vi "vision board process.vi"(11 "Array in":string[][](array[string])) -> (3 "Array out":string[][](array[string]))   [LabVIEW 2019]
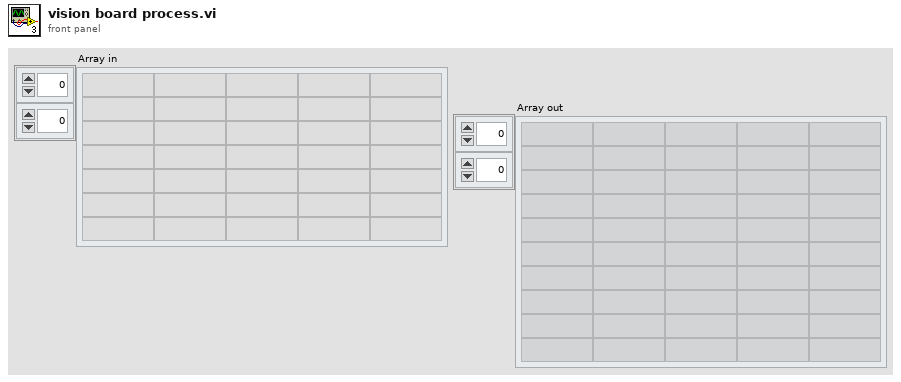
[diagram p1: front panel]
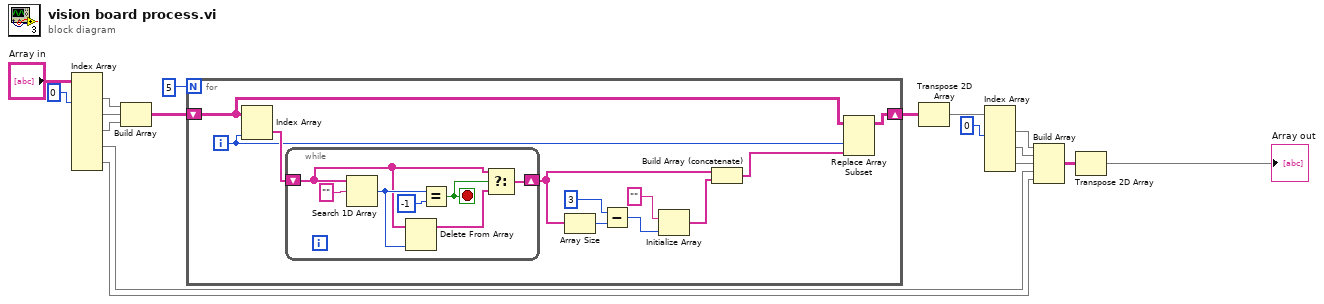
[diagram p0: block diagram]
diagram:
  n1 = Index Array(array="Array in", index (col) #1=0 ("disabled index (col)")) -> (element #1=w1:string[], element #2=w3:string[], element #3=w2:string[], element #4=w13:string[], element #5=w12:string[])  [unwired: 9 in]
  n2 = Build Array(w1, w3, w2) -> (w6:string[][])
  n3 = for {
    N: 5 -> [_]
    shift-right: [w28] -> w11
    shift-left: w6 -> [w26]
    i -> [w25]
    n4 = Index Array(array=w26, index (col)=w25) -> (element=w27:string[])  [unwired: 1 in]
    n5 = while {
      shift-right: [w29] -> w19
      shift-left: w27 -> [w30]
      stop <- w31 stop-if-true
      n6 = Search 1D Array(1D array=w30, element="") -> (index of element=w33:i32)  [unwired: 1 in]
      n7 = Delete From Array(array=w30, index=w33) -> (array with subset deleted=w32:string[])  [unwired: 1 in, 1 out]
      n8 = Equal?(x=w33, y=-1) -> (x = y?=w31:bool)
      n9 = Select(t=w30, s=w31, f=w32) -> (s? t:f=w29:string[])
    }
    n10 = Array Size(array=w19) -> (size(s)=w23:i32)
    n11 = Subtract(x=3, y=w23) -> (x-y=w21:i32)
    n12 = Initialize Array("", w21) -> (w20:string[])
    n13 = Build Array (concatenate)(w19, w20) -> (w18:string[])
    n14 = Replace Array Subset(array=w26, new element=w18, index (col)=w25) -> (w28:string[][])  [unwired: 1 in]
  }
  n15 = Transpose 2D Array(2D array=w11) -> (transposed array=w16:string[][])
  n16 = Index Array(array=w16, index (col) #1=0 ("index (col)")) -> (element #1=w9:string[], element #2=w7:string[], element #3=w8:string[])  [unwired: 5 in]
  n17 = Build Array(w9, w7, w8, w13, w12) -> (w14:string[][])
  n18 = Transpose 2D Array(2D array=w14) -> (transposed array=→"Array out":string[][])
